vi "Close Events.vi"(11 "events":refnum<event-registration>) -> ()   [LabVIEW 2014, in "Observable Actor.lvlib" / "Observable Actor.lvclass"]
uses:
  Observable Actor.lvclass
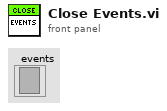
[diagram p1: front panel]
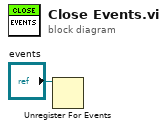
[diagram p0: block diagram]
diagram:
  n1 = Unregister For Events(event registration refnum="events") -> ()  [unwired: 1 in, 1 out]
